vi "FL_Align_and_Decode_input_data.vi"(9 "Input timestamp":timestamp, 10 "Input string in":string, 11 "SB size (loc. var. only)":u8) -> (2 "DEC output cluster":T1, 3 "Input string out":string)   [LabVIEW 2018, in "Tracker.lvlib"]
uses:
  Tracker.lvlib
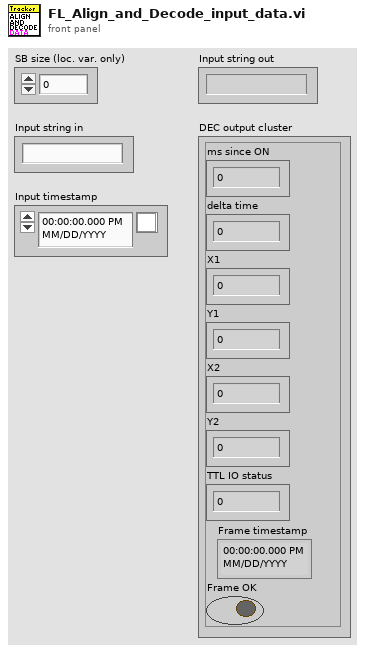
[diagram p1: front panel]
types:
  T1 = cluster{"ms since ON":u32, "delta time":u32, "X1":sgl, "Y1":sgl, "X2":sgl, "Y2":sgl, "TTL IO status":u8, "Frame timestamp":timestamp, "Frame OK":bool}
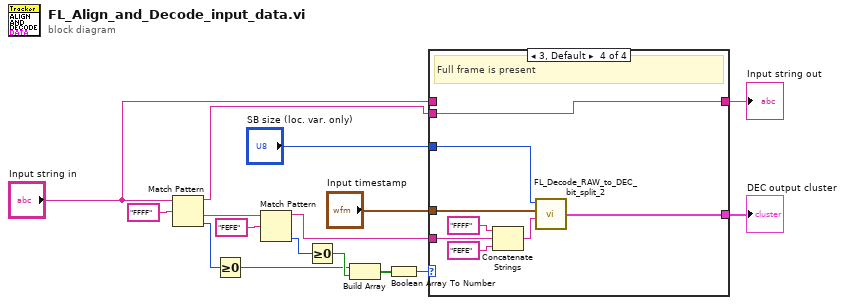
[diagram p0: block diagram]
diagram:
  n1 = Match Pattern(string="Input string in", regular expression="FFFF") -> (before substring=w13:string, after substring=w12:string, offset past match=w8:i32)  [unwired: 1 in, 1 out]
  n2 = Greater Or Equal To 0?(x=w8) -> (x >= 0?=w3:bool)
  n3 = Match Pattern(string=w12, regular expression="FEFE") -> (before substring=w9:string, offset past match=w7:i32)  [unwired: 1 in, 2 out]
  n4 = Greater Or Equal To 0?(x=w7) -> (x >= 0?=w4:bool)
  n5 = Build Array(w3, w4) -> (w6:bool[])
  n6 = Boolean Array To Number(Boolean array=w6) -> (number=w5:u32)
  n7 = case shown="3, Default" w5 {
    tunnel: w9 -> [_ _ _ w26]
    tunnel: [_ _ _ w27] -> w15
    tunnel: "Input timestamp" -> [_ _ _ w21]
    tunnel: [w17 w18 w19 w22] -> w11
    tunnel: w13 -> [_ _ _ w22]
    tunnel: "Input string in" -> [w17 w18 w19 _]
    tunnel: "SB size (loc. var. only)" -> [_ _ _ w20]
    frame 0 {
      # "Neither beginning, nor ending of frame is present"
    }
    frame 1 {
      # "Only frame beginning is present"
    }
    frame 2 {
      # "Only frame end is present"
    }
    frame 3, Default {
      # "Full frame is present"
      n8 = Concatenate Strings("FFFF" ("string"), w26, "FEFE" ("string")) -> (w25:string)
      n9 = call "FL_Decode_RAW_to_DEC_bit_split_2.vi"("Read buffer text to decode"=w25, "Input timestamp"=w21, "SB size (loc. var. only)"=w20) -> ("DEC output cluster"=w27:T1)  [unwired: 1 in]
    }
  }
  "DEC output cluster" <- w15
  "Input string out" <- w11
